vi "GetDefaultConfigFilePath.vi"() -> ()   [LabVIEW 2020]
panel:
  out "XML File Path":path
  out "error out":errorcluster
  in  "error in (no error)":errorcluster
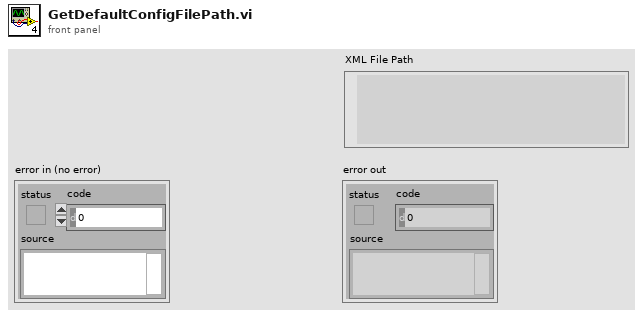
[diagram p1: front panel]
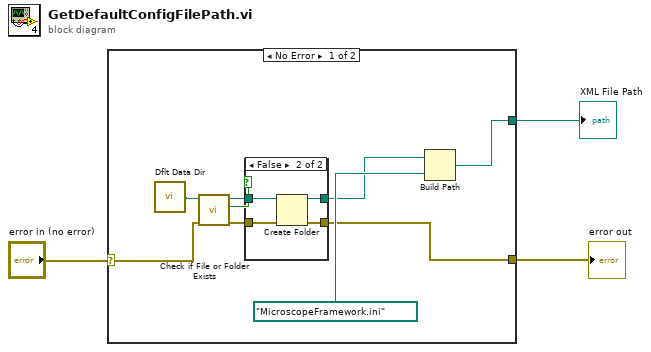
[diagram p0: block diagram]
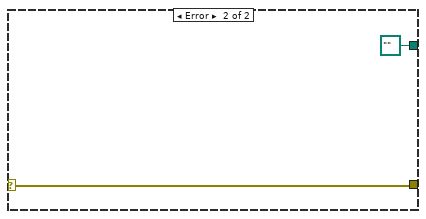
[diagram p3: hidden frame]
diagram:
  n1 = case shown="No Error" "error in (no error)" {
    selector: "error in (no error)" -> [w5 w19]
    tunnel: [w11 path "" ("appended path")] -> w3
    tunnel: [w4 w19] -> w1
    frame No Error {
      n2 = call <vilib>:"Dflt Data Dir.vi"() -> ("App:Default Data Directory"=w7:path)
      n3 = call <vilib>:"Check if File or Folder Exists.vi"("error in (no error)"=w5, "path"=w7) -> ("error out"=w9:errorcluster, "file or folder exists?"=w8:bool, "dup path"=w10:path)  [unwired: 7 in]
      n4 = case shown="False" w8 {
        tunnel: w9 -> [w13 w18]
        tunnel: w10 -> [w14 w17]
        tunnel: [w13 w16] -> w4
        tunnel: [w14 w15] -> w6
        frame True {
        }
        frame False {
          n5 = Create Folder(path (use dialog)=w17, error in=w18) -> (created path=w15:path, error out=w16:errorcluster)  [unwired: 1 in, 1 out]
        }
      }
      n6 = Build Path(base path=w6, name or relative path=path "MicroscopeFramework.ini" ("string")) -> (appended path=w11:path)
    }
    frame Error {
    }
  }
  "error out" <- w1
  "XML File Path" <- w3
